vi "Report for Internal EEPROM.vi"(8 "Error":string, 9 "Pass?":bool, 10 "EEPROM contents":string="¯õZ¬€\u0000\"PZý4\u0019a–ÿÿÿBL 6331 V1.01       104  LCU 6330/6331     \u0000", 11 "Time Stamp":timestamp) -> (3 "Report Body":string)   [LabVIEW 2009]
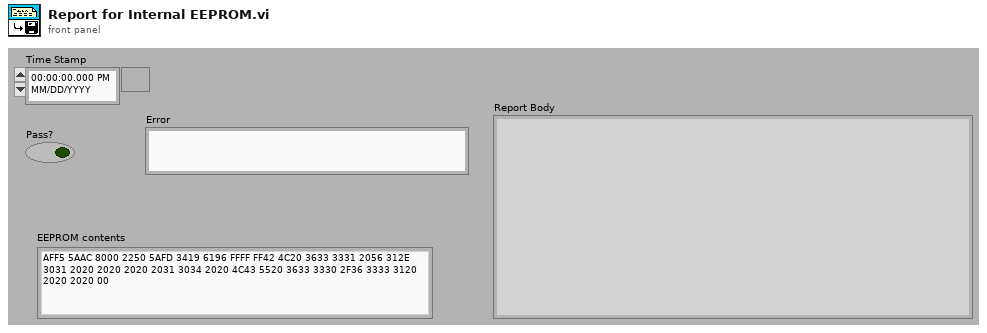
[diagram p1: front panel]
types:
  T1 = typedef "LVDateTimeRec.ctl" = cluster{"fractional second":dbl, "second":i32, "minute":i32, "hour":i32, "day of month":i32, "month":i32, "year":i32, "day of week":i32, "day of year":i32, "DST":i32}
  T2 = cluster{"year":i32, "month":i32, "day of month":i32, "hour":i32, "minute":i32, "second":i32}
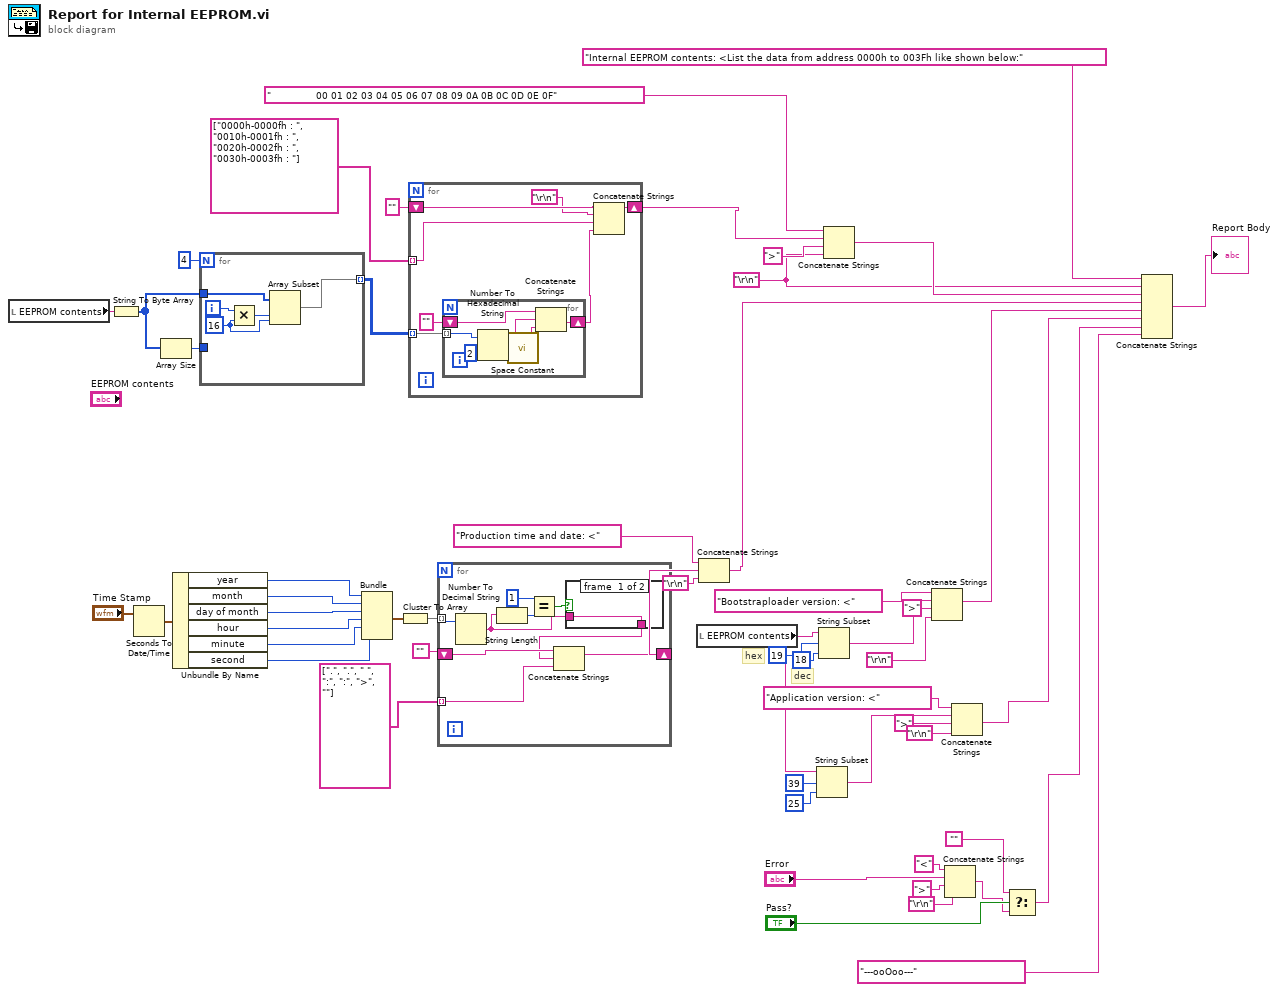
[diagram p0: block diagram]
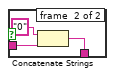
[diagram p2: hidden frame]
diagram:
  w6 = "\r\n"
  # "dec"
  # "hex"
  n1 = local read "EEPROM contents"() -> (w54:string)
  n2 = String To Byte Array(string=w54) -> (unsigned byte array=w45:u8[])
  n3 = Seconds To Date/Time(time stamp (now)="Time Stamp") -> (date time rec=w44:T1)  [unwired: 1 out]
  n4 = Array Size(array=w45) -> (size(s)=w53:i32)
  n5 = Unbundle By Name(w44) -> ("year"=w43:i32, "month"=w42:i32, "day of month"=w41:i32, "hour"=w40:i32, "minute"=w35:i32, "second"=w39:i32)
  n6 = for {
    N: 4 -> [_]
    tunnel: w45 -> [w58]
    tunnel: [w56] -> w52 mode=indexing
    tunnel: w53 -> [_]
    i -> [w59]
    w57 = 16 ("y")
    n7 = Multiply(x=w59, y=w57) -> (x*y=w55:i32)
    n8 = Array Subset(array=w58, index=w55, length=w57) -> (w56:u8[])
  }
  n9 = Bundle("year"=w43, "month"=w42, "day of month"=w41, "hour"=w40, "minute"=w35, "second"=w39) -> (w38:T2)  [unwired: 1 out]
  n10 = Cluster To Array(cluster=w38) -> (array=w37:i32[])
  n11 = for {
    tunnel: w52 -> [w66] mode=indexing
    tunnel: string[] ["0000h-0000fh : ", "0010h-0001fh : ", "0020h-0002fh : ", "0030h-0003fh : "] ("Array 2") -> [w64] mode=indexing
    shift-right: [w62] -> w48
    shift-left: "" -> [w61]
    n12 = for {
      tunnel: w66 -> [w72] mode=indexing
      shift-right: [w68] -> w63
      shift-left: "" -> [w70]
      n13 = Number To Hexadecimal String(1:i16 2 ("width (-)"), 2:w72) -> (0:w69:string)
      n14 = call <vilib>:"Space Constant.vi"() -> ("String"=w67:string)
      n15 = Concatenate Strings(w70, w69, w67) -> (w68:string)
    }
    n16 = Concatenate Strings(w61, "\r\n", w64, w63) -> (w62:string)
  }
  n17 = for {
    tunnel: w37 -> [w81] mode=indexing
    shift-right: [w79] -> w32
    shift-left: "" -> [w80]
    tunnel: string[] [".", ".", " ", ":", ":", ">", ""] -> [w78] mode=indexing
    n18 = Number To Decimal String(number=w81) -> (decimal integer string=w74:string)  [unwired: 1 out]
    n19 = String Length(string=w74) -> (length=w77:i32)
    n20 = Equal?(x=1, y=w77) -> (x = y?=w75:bool)
    n21 = case shown="False" w75 {
      tunnel: w74 -> [w82 w85]
      tunnel: [w82 w83] -> w73
      frame #0 {
      }
      frame #1 {
        n22 = Concatenate Strings("0" ("string"), w85) -> (w83:string)
      }
    }
    n23 = Concatenate Strings(w80, w73, w78) -> (w79:string)
  }
  n24 = local read "EEPROM contents"() -> (w24:string)
  n25 = Concatenate Strings("Production time and date: <" ("string"), w32, "\r\n") -> (w5:string)
  n26 = String Subset(string=w24, offset (0)=39, length (rest)=25 ("offset (0)")) -> (substring=w21:string)
  n27 = String Subset(string=w24, offset (0)=19, length (rest)=18 ("offset (0)")) -> (substring=w28:string)
  n28 = Concatenate Strings("               00 01 02 03 04 05 06 07 08 09 0A 0B 0C 0D 0E 0F" ("string"), w48, ">" ("string"), w6) -> (w13:string)
  n29 = Concatenate Strings("Bootstraploader version: <" ("string"), w28, ">" ("string"), "\r\n") -> (w12:string)
  n30 = Concatenate Strings("<" ("string"), "Error", ">" ("string"), "\r\n") -> (w1:string)
  n31 = Concatenate Strings("Application version: <" ("string"), w21, ">" ("string"), "\r\n") -> (w11:string)
  n32 = Select(t="", s="Pass?", f=w1) -> (s? t:f=w10:string)
  n33 = Concatenate Strings("Internal EEPROM contents: <List the data from address 0000h to 003Fh like shown below:" ("string"), w6, w13, w5, w12, w11, w10, "---ooOoo---" ("string")) -> (→"Report Body":string)
